vi "OpenGDSLicense_ProductInfo.vi"(5 "error in (no error)":errorcluster) -> (19 "error out":errorcluster)   [LabVIEW 2012]
uses:
  <resource>/Framework/Providers/Open_GDS/ClassProviders/Provider_EndevoGOOP300/ClassWriterGOOP300_class/ClassWriterGOOP300.lvclass
  <resource>/Framework/Providers/Open_GDS/ClassProviders/Provider_LvNativeClass/ClassWriterNative_class/ClassWriterNative.lvclass
  <resource>/Framework/Providers/Open_GDS/ClassProviders/Provider_EndevoGOOP400/ClassWriterGOOP400_class/ClassWriterGOOP400.lvclass
  <vilib>/event_ctls.llb/lveventtype.ctl
  <resource>/Framework/Providers/Open_GDS/SubVIs/GOOP_ToolVersion.vi
  <vilib>/Platform/browser.llb/Open URL in Default Browser (string).vi
panel:
  out "SwCheck":string
  in  "_GDSOnline":bool
  in  "_MainHelp":bool
  in  "_UnInstall":bool
  out "_Version":string="4.1  (Q3U)" caption="Version"
  in  "_OK":bool
  # "Open GOOP\nDevelopment Suite"
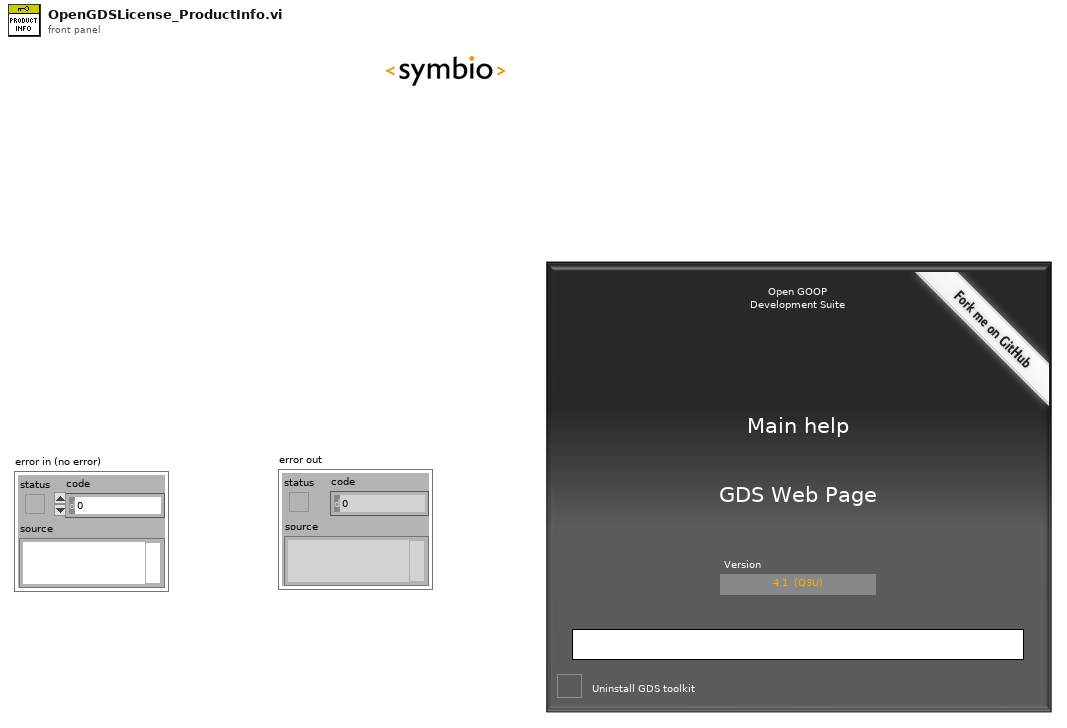
[diagram p1: front panel]
types:
  T1 = cluster{"Templates":path[], "TemplatesVersions":string[], "KernelVIs":path[], "KernelVersions":string[]}
  T2 = enum32{"None", "Stop", "Question", "Exclamation", "Information"}
  T3 = typedef "lveventtype.ctl" = enum32{"Null", "Timeout", "Annotation Menu Selection", "Annotation Menu Selection?", "App Instance Close", "App Instance Close?", "Autoscale Range Change", "Cell Edit", "Cell Edit?", "Cursor Grab", "Cursor Grab?", "Cursor Menu Selection", "Cursor Menu Selection?", "Cursor Move", "Cursor Release", "Data Change", "Direction Change", "Display State Change", "Drag Ended", "Drag Enter", "Drag Leave", "Drag Over", "Drag Source Update", "Drag Starting", "Drag Starting?", "Drop", "Exec State Change", "Key Down", "Key Down?", "Key Repeat", "Key Repeat?", "Key Up", "Listbox Double Click", "Menu Activation?", "Menu Selection (App)", "Menu Selection? (App)", "Menu Selection (User)", "Mouse Down", "Mouse Down?", "Mouse Enter", "Mouse Leave", "Mouse Move", "Mouse Up", "NI Security User Change (App)", "Pane Size", "Panel Close", "Panel Close?", "Panel Resize", "Plot Attribute Change", "Scale Range Change", "Shortcut Menu Activation?", "Shortcut Menu Selection (App)", "Shortcut Menu Selection? (App)", "Shortcut Menu Selection (User)", "Tree Double Click", "Tree Drag", "Tree Drag?", "Tree Drop", "Tree Drop?", "Tree Item Close", "Tree Item Close?", "Tree Item Open", "Tree Item Open?", "Value Change"}
  T4 = cluster{"Major":u16, "Minor":u16, "Fix":u16, "Build":u16}
  T5 = typedef "Librarian File List.ctl" = cluster{"name":string, "create date":u32, "mod date":u32, "type":string, "creator":string, "LV version":i32}[]
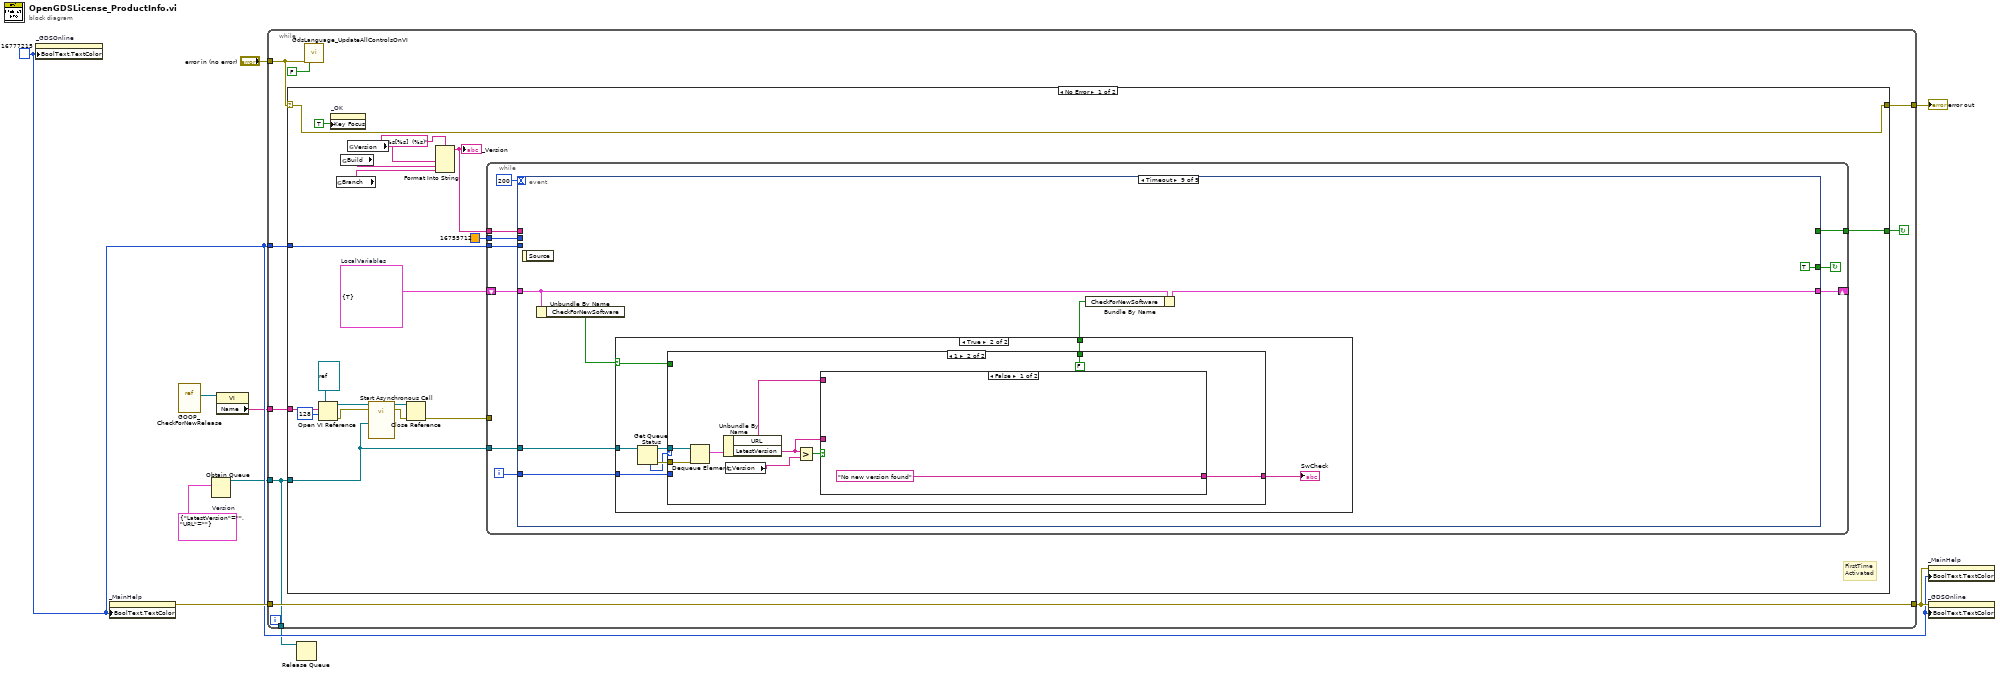
[diagram p0: block diagram]
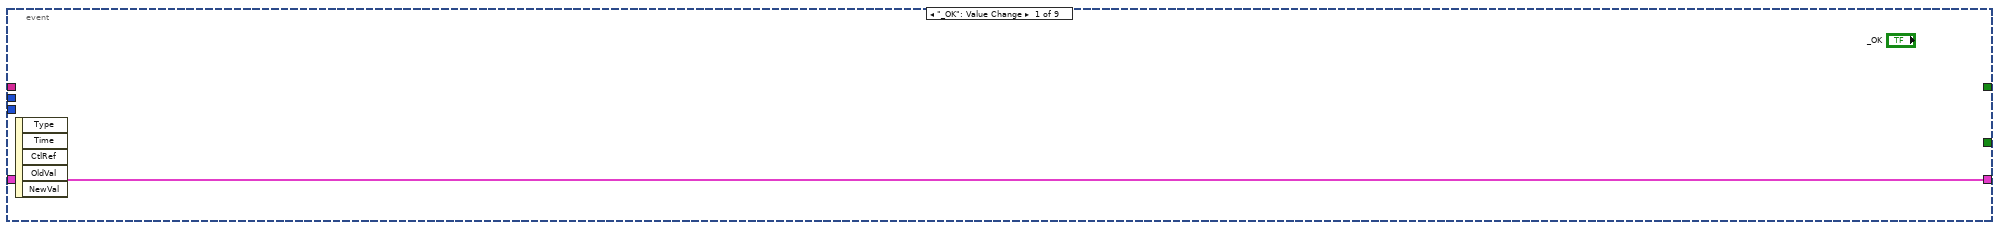
[diagram p2: hidden frame]
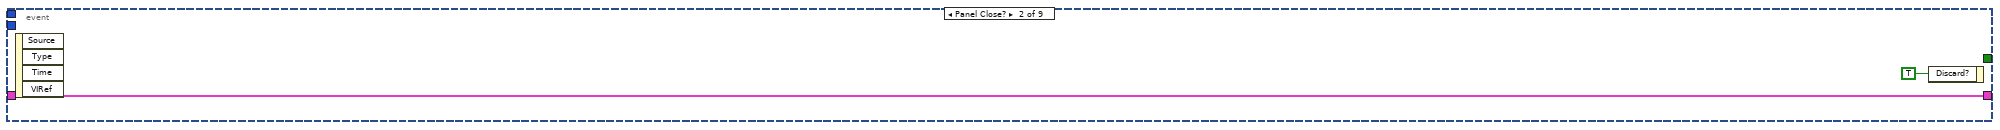
[diagram p3: hidden frame]
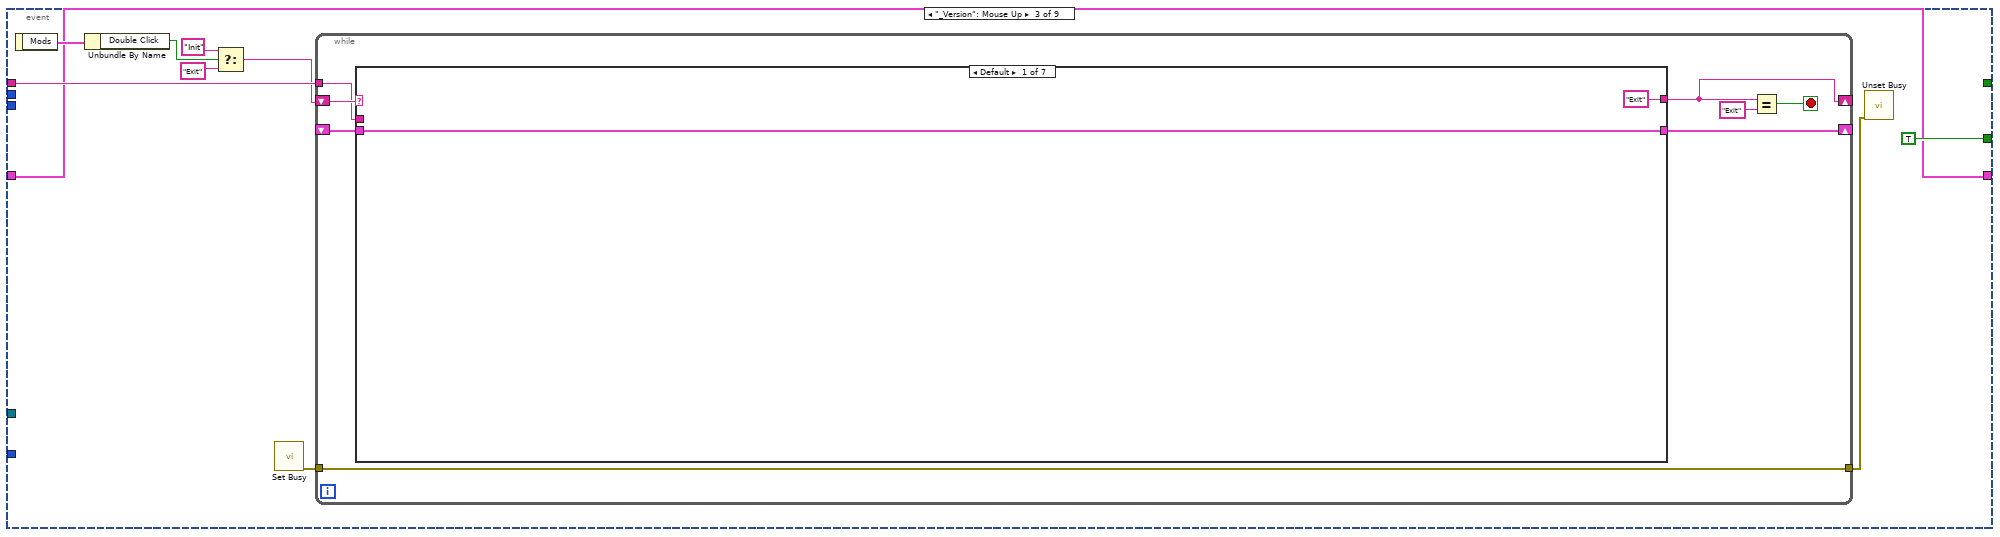
[diagram p4: hidden frame]
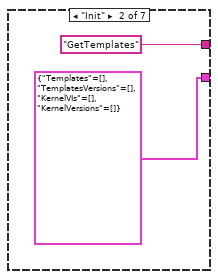
[diagram p5: hidden frame]
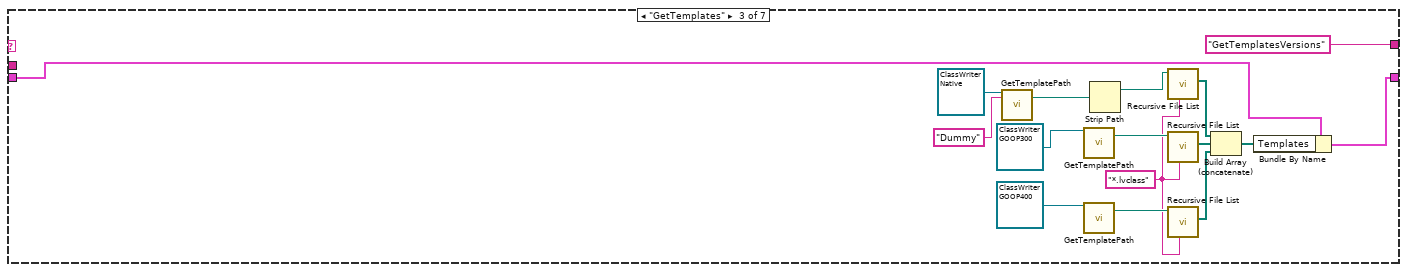
[diagram p6: hidden frame]
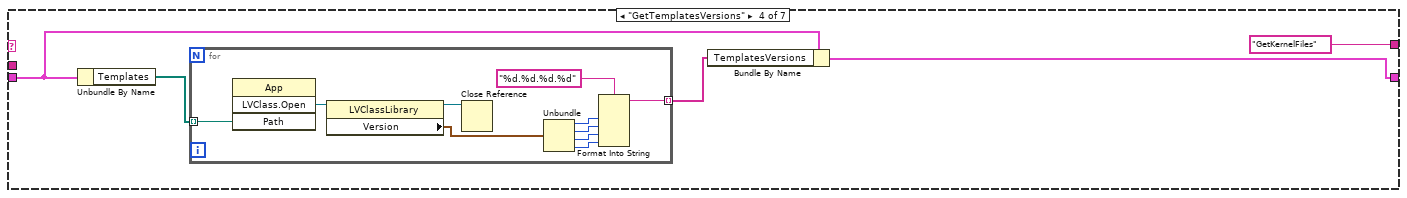
[diagram p7: hidden frame]
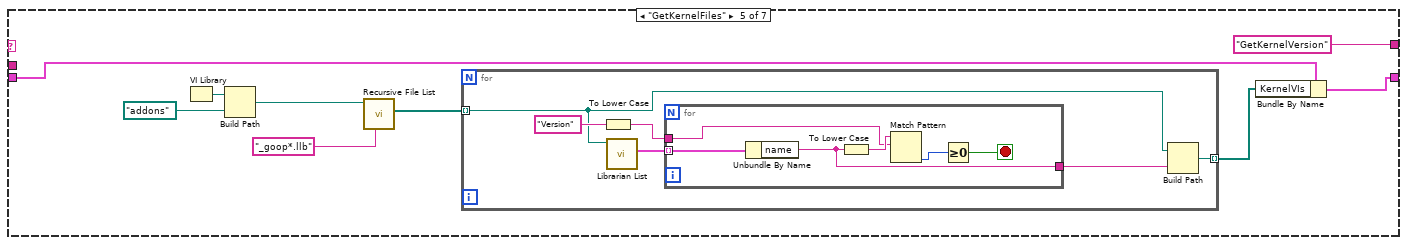
[diagram p8: hidden frame]
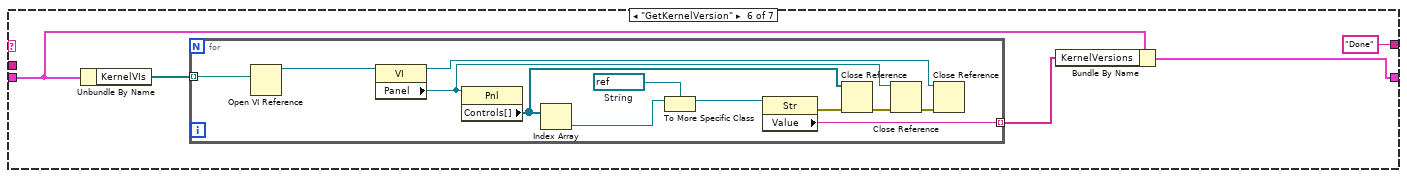
[diagram p9: hidden frame]
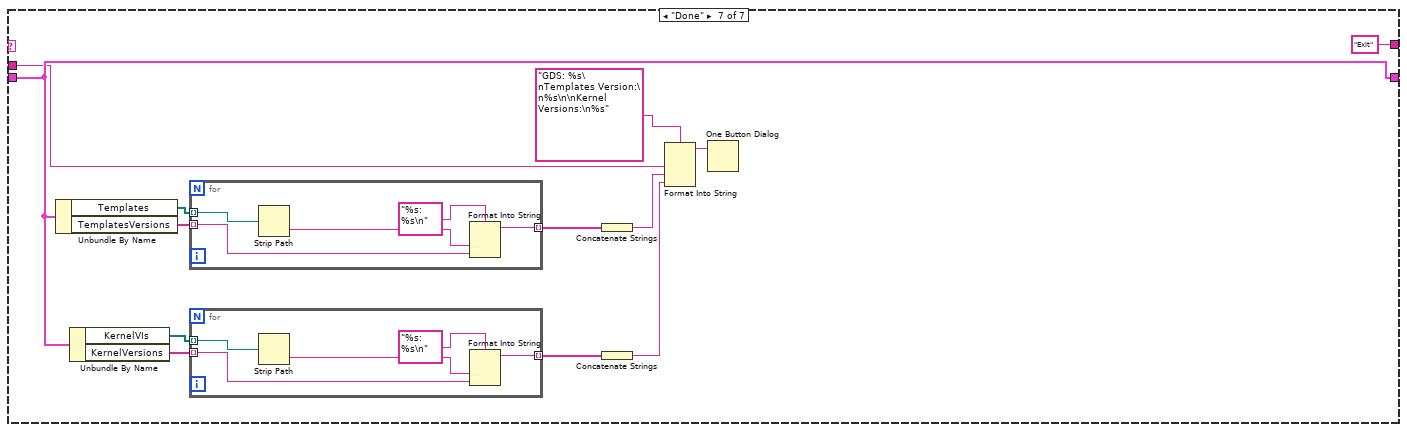
[diagram p10: hidden frame]
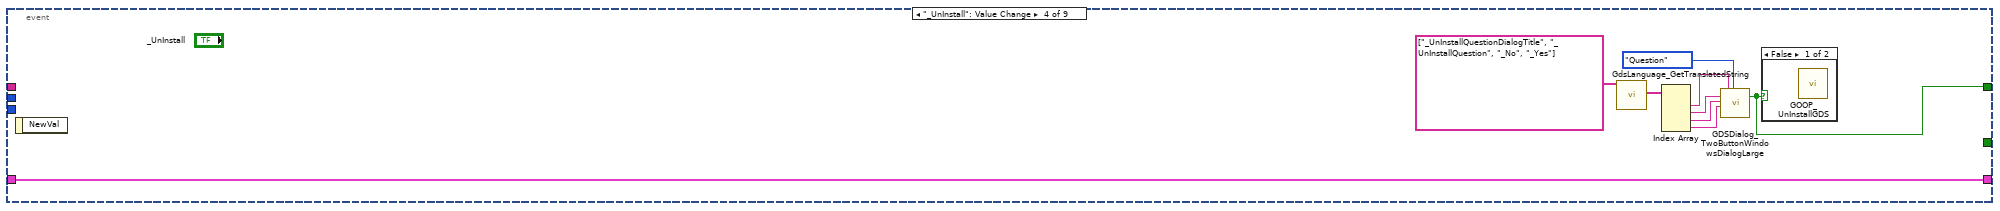
[diagram p11: hidden frame]
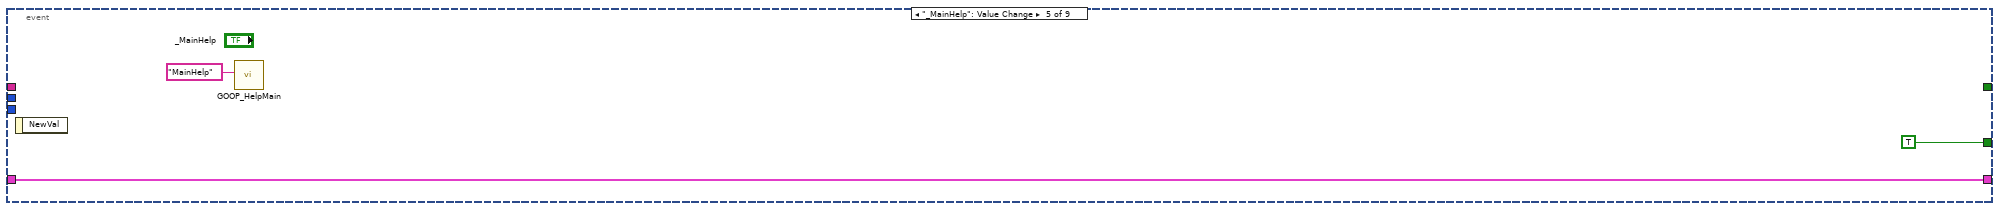
[diagram p13: hidden frame]
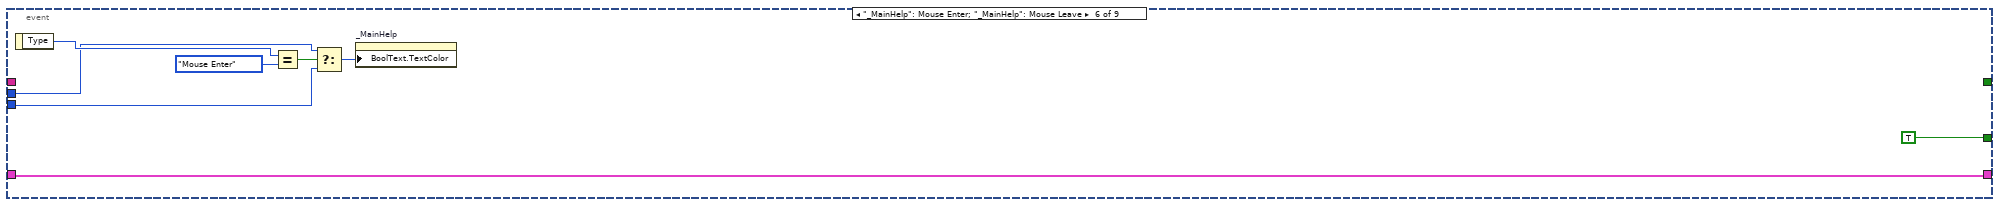
[diagram p14: hidden frame]
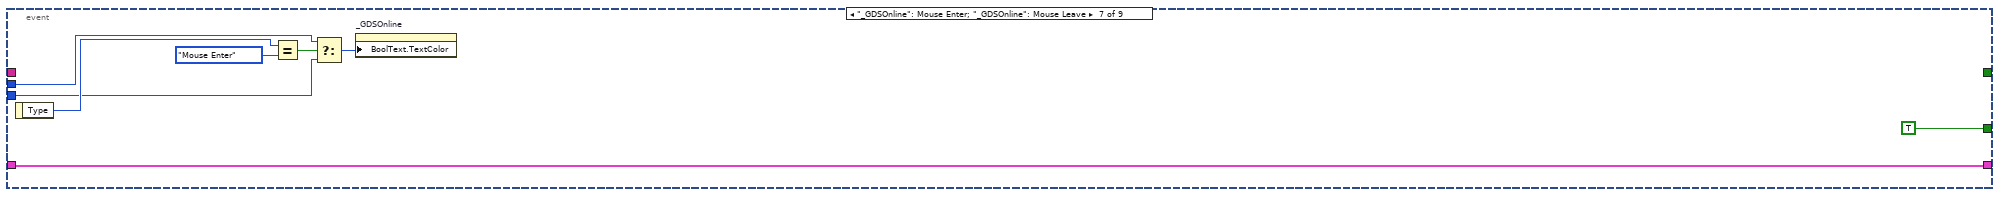
[diagram p15: hidden frame]
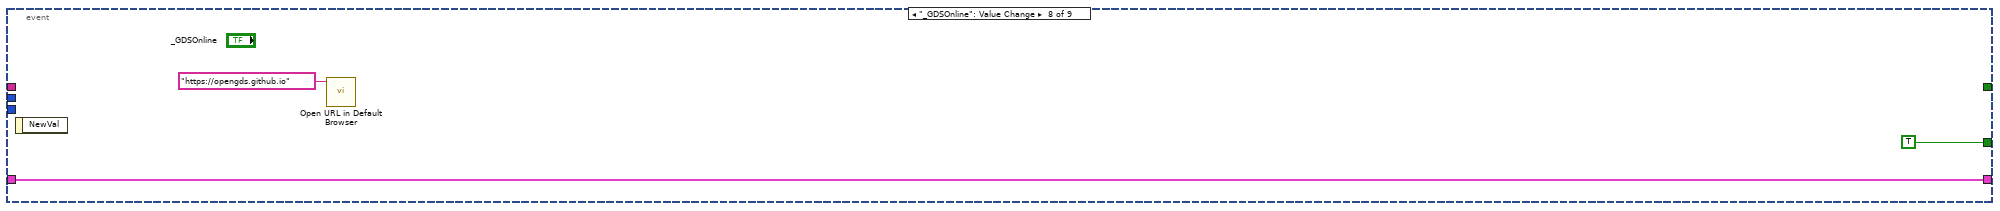
[diagram p16: hidden frame]
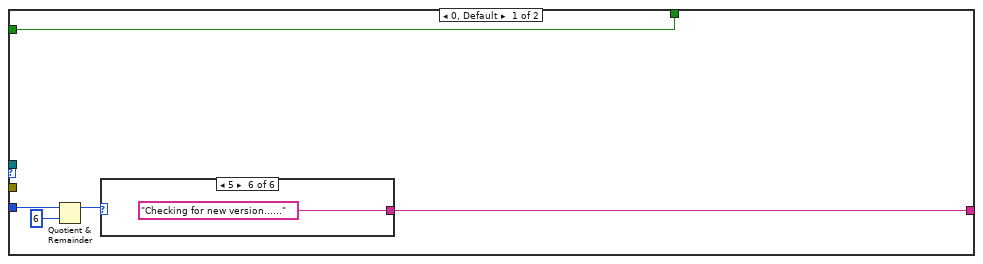
[diagram p18: hidden frame]
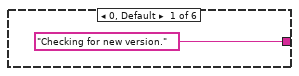
[diagram p19: hidden frame]
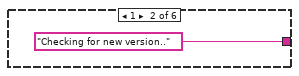
[diagram p20: hidden frame]
diagram:
  w3 = cluster{"LatestVersion":string, "URL":string} {"LatestVersion"="", "URL"=""}  # Version
  w6 = u32 16777215
  n1 = property on="_GDSOnline" class="Bool"("BoolText.TextColor"=w6) -> ()  [unwired: 2 in, 2 out]
  n2 = property on="_MainHelp" class="Bool"("BoolText.TextColor"=w6) -> (error out=w8:errorcluster)  [unwired: 2 in, 1 out]
  n3 = vi-ref <resource>:"GOOP_CheckForNewRelease.vi"() -> (w5:refnum<vi>)
  n4 = Obtain Queue(element data type=w3) -> (queue out=w2:refnum<queue>)  [unwired: 4 in, 2 out]
  n5 = property class="VI"(reference=w5) -> ("Name"=w4:string)  [unwired: 1 in, 2 out]
  n6 = while {
    tunnel: [w18] -> w10
    tunnel: "error in (no error)" -> [w13]
    tunnel: [w15] -> w7
    tunnel: w8 -> [w15]
    tunnel: w6 -> [w14]
    tunnel: w4 -> [w12]
    tunnel: w2 -> [w11]
    tunnel: [w11] -> w1
    stop <- w16 continue-if-true
    n7 = case shown="No Error" w13 {
      selector: w13 -> [w38 w244]
      tunnel: [w38 w244] -> w18
      tunnel: [w37 _] -> w16
      tunnel: w14 -> [w36 _]
      tunnel: w12 -> [w30 _]
      tunnel: w11 -> [w21 _]
      frame No Error {
        w26 = cluster{"CheckForNewSoftware":bool} {"CheckForNewSoftware"=TRUE}  # LocalVariables
        # "FirstTime\nActivated"
        n8 = Open VI Reference(type specifier VI Refnum (for type only)=refnum<vi> refnum, vi path=w30, options=128) -> (vi reference=w29:refnum<vi>, error out=w28:errorcluster)  [unwired: 3 in]
        n9 = property on="_OK" class="Bool"("Key Focus"=TRUE) -> ()  [unwired: 2 in, 2 out]
        n10 = global read "GOOP_ToolVersion.vi" "Branch"() -> (w20:string)
        n11 = global read "GOOP_ToolVersion.vi" "Build"() -> (w19:string)
        n12 = global read "GOOP_ToolVersion.vi" "Version"() -> (w35:string)
        n13 = call-by-ref "Start Asynchronous Call"(reference=w29, error in=w28, "QueueRef"=w21) -> (reference out=w24:refnum<vi>, error out=w23:errorcluster)  [unwired: 11 in]
        n14 = Close Reference(reference=w24, error in (no error)=w23) -> (error out=w22:errorcluster)
        n15 = Format Into String(format string="%s[%s]  (%s)", w35, w19, w20) -> (resulting string=w33:string)  [unwired: 2 in, 1 out]
        "_Version" <- w33
        n16 = while {
          tunnel: [w48] -> w37
          tunnel: w33 -> [w47]
          tunnel: u32 16755712 -> [w45]
          tunnel: w36 -> [w44]
          shift-right: [w41] -> _
          shift-left: w26 -> [w42]
          tunnel: w21 -> [w40]
          tunnel: w22 -> [_]
          i -> [w39]
          stop <- w46 continue-if-true
          n17 = event shown="[8] Timeout" {
            selector: _ -> [_ _ _ _ _ _ _ _ _]
            dyn-events: _ -> [_ _ _ _ _ _ _ _ _]
            timeout: 200 -> [_ _ _ _ _ _ _ _ _]
            tunnel: [_ _ _ w167 _ _ _ _ _] -> w48
            tunnel: w47 -> [_ _ w58 _ _ _ _ _ _]
            tunnel: [_ _ TRUE _ TRUE TRUE TRUE TRUE TRUE] -> w46
            tunnel: w45 -> [_ _ _ _ _ w180 w188 _ _]
            tunnel: w44 -> [_ _ _ _ _ w179 w187 _ _]
            tunnel: w42 -> [w49 w50 w52 w166 w175 w178 w186 w194 w203]
            tunnel: [w49 w50 w52 w166 w175 w178 w186 w194 w198] -> w41
            tunnel: w40 -> [_ _ _ _ _ _ _ _ w201]
            tunnel: w39 -> [_ _ _ _ _ _ _ _ w200]
            event "_OK": Value Change {
              n18 = event-data() -> ()  [unwired: 1 in, 5 out]
            }
            event Panel Close? {
              n19 = event-data() -> ()  [unwired: 1 in, 4 out]
              n20 = event-data("Discard?"=TRUE) -> ()  [unwired: 1 in, 1 out]
            }
            event "_Version": Mouse Up {
              n21 = event-data() -> ("Mods"=w61:cluster{"Double Click":bool, "Menu Key":bool})  [unwired: 1 in]
              n22 = Unbundle By Name(w61) -> ("Double Click"=w57:bool)
              n23 = Select(t="Init", s=w57, f="Exit") -> (s? t:f=w54:string)
              n24 = call <vilib>:"Set Busy.vi"() -> ("error out"=w60:errorcluster)  [unwired: 10 in, 1 out]
              n25 = while {
                shift-right: [w64] -> _
                shift-left: w54 -> [w69]
                shift-right: [w66] -> _
                shift-left: _ -> [w65]
                tunnel: w60 -> [w63]
                tunnel: [w63] -> w59
                tunnel: w58 -> [w62]
                stop <- w68 stop-if-true
                n26 = case shown="Default" w69 {
                  tunnel: ["Exit" "GetTemplates" "GetTemplatesVersions" "GetKernelFiles" "GetKernelVersion" "Done" "Exit"] -> w64
                  tunnel: [w70 T1 {"Templates"=[], "TemplatesVersions"=[], "KernelVIs"=[], "KernelVersions"=[]} w83 w91 w106 w127 w145] -> w66
                  tunnel: w65 -> [w70 _ w84 w93 w108 w129 w145]
                  tunnel: w62 -> [_ _ _ _ _ _ w143]
                  frame Default {
                  }
                  frame "Init" {
                  }
                  frame "GetTemplates" {
                    w77 = "*.lvclass" ("pattern")
                    n27 = call-dynamic "GetTemplatePath.vi"("reference in"=refnum<class "ClassWriterNative.lvclass"> refnum, "ClassTemplateSubDirectory"="Dummy") -> ("FolderPathOut"=w75:path)  [unwired: 14 in, 3 out]
                    n28 = call-dynamic "GetTemplatePath.vi"("reference in"=refnum<class "ClassWriterGOOP300.lvclass"> refnum) -> ("FolderPathOut"=w82:path)  [unwired: 15 in, 3 out]
                    n29 = call-dynamic "GetTemplatePath.vi"("reference in"=refnum<class "ClassWriterGOOP400.lvclass"> refnum ("ClassWriterGOOP400.lvclass")) -> ("FolderPathOut"=w80:path)  [unwired: 15 in, 3 out]
                    n30 = Strip Path(path=w75) -> (stripped path=w74:path)  [unwired: 1 out]
                    n31 = call <vilib>:"Recursive File List.vi"("pattern"=w77, "Folder Path"=w74) -> ("All Files in Dir"=w86:path[])  [unwired: 5 in, 4 out]
                    n32 = call <vilib>:"Recursive File List.vi"("pattern"=w77, "Folder Path"=w82) -> ("All Files in Dir"=w81:path[])  [unwired: 5 in, 4 out]
                    n33 = call <vilib>:"Recursive File List.vi"("pattern"=w77, "Folder Path"=w80) -> ("All Files in Dir"=w79:path[])  [unwired: 5 in, 4 out]
                    n34 = Build Array (concatenate)(w86, w81, w79) -> (w85:path[])
                    n35 = Bundle By Name(cluster=w84, "Templates"=w85) -> (w83:T1)
                  }
                  frame "GetTemplatesVersions" {
                    n36 = Unbundle By Name(w93) -> ("Templates"=w94:path[])
                    n37 = for {
                      tunnel: w94 -> [w104] mode=indexing
                      tunnel: [w96] -> w92 mode=indexing
                      n38 = invoke class="App" method="LVClass.Open"("Path"=w104) -> ("LVClass.Open"=w103:refnum<vi>)  [unwired: 3 in, 3 out]
                      n39 = property class="LVClassLibrary"(reference=w103) -> (reference out=w95:refnum<vi>, "Version"=w102:T4)  [unwired: 1 in, 1 out]
                      n40 = Close Reference(reference=w95) -> ()  [unwired: 1 in, 1 out]
                      n41 = Unbundle(w102) -> ("Major"=w100:u16, "Minor"=w99:u16, "Fix"=w98:u16, "Build"=w97:u16)
                      n42 = Format Into String(format string="%d.%d.%d.%d", w100, w99, w98, w97) -> (resulting string=w96:string)  [unwired: 2 in, 1 out]
                    }
                    n43 = Bundle By Name(cluster=w93, "TemplatesVersions"=w92) -> (w91:T1)
                  }
                  frame "GetKernelFiles" {
                    n44 = VI Library() -> (path=w113:path)
                    n45 = Build Path(base path=w113, name or relative path=path "addons") -> (appended path=w111:path)
                    n46 = call <vilib>:"Recursive File List.vi"("pattern"="_goop*.llb", "Folder Path"=w111) -> ("All Files in Dir"=w109:path[])  [unwired: 5 in, 4 out]
                    n47 = for {
                      tunnel: w109 -> [w115] mode=indexing
                      tunnel: [w114] -> w107 mode=indexing
                      n48 = To Lower Case(string="Version" ("regular expression")) -> (all lower case string=w117:string)
                      n49 = call <vilib>:"Librarian List.vi"("path"=w115) -> ("file list"=w119:T5)  [unwired: 9 in, 1 out]
                      n50 = for {
                        tunnel: w119 -> [w125] mode=indexing
                        tunnel: w117 -> [w123]
                        tunnel: [w120] -> w116
                        stop <- w121 stop-if-true
                        n51 = Unbundle By Name(w125) -> ("name"=w120:string)
                        n52 = To Lower Case(string=w120) -> (all lower case string=w124:string)
                        n53 = Match Pattern(string=w124, regular expression=w123) -> (offset past match=w122:i32)  [unwired: 1 in, 3 out]
                        n54 = Greater Or Equal To 0?(x=w122) -> (x >= 0?=w121:bool)
                      }
                      n55 = Build Path(base path=w115, name or relative path=w116) -> (appended path=w114:path)
                    }
                    n56 = Bundle By Name(cluster=w108, "KernelVIs"=w107) -> (w106:T1)
                  }
                  frame "GetKernelVersion" {
                    n57 = Unbundle By Name(w129) -> ("KernelVIs"=w130:path[])
                    n58 = for {
                      tunnel: w130 -> [w142] mode=indexing
                      tunnel: [w137] -> w128 mode=indexing
                      w139 = refnum<vi> refnum  # String
                      n59 = Open VI Reference(vi path=w142) -> (vi reference=w141:refnum<vi>)  [unwired: 5 in, 1 out]
                      n60 = property class="VI"(reference=w141) -> (reference out=w131:refnum<vi>, "Panel"=w133:refnum<vi>)  [unwired: 1 in, 1 out]
                      n61 = property class="Pnl"(reference=w133) -> ("Controls[]"=w135:refnum<vi>[])  [unwired: 1 in, 2 out]
                      n62 = Index Array(array=w135) -> (element=w140:refnum<vi>)  [unwired: 1 in]
                      n63 = To More Specific Class(target class=w139, reference=w140) -> (specific class reference=w138:refnum<vi>)  [unwired: 1 in, 1 out]
                      n64 = property class="Str"(reference=w138) -> (error out=w136:errorcluster, "Value"=w137:string)  [unwired: 1 in, 1 out]
                      n65 = Close Reference(reference=w135, error in (no error)=w136) -> (error out=w134:errorcluster)
                      n66 = Close Reference(reference=w133, error in (no error)=w134) -> (error out=w132:errorcluster)
                      n67 = Close Reference(reference=w131, error in (no error)=w132) -> ()  [unwired: 1 out]
                    }
                    n68 = Bundle By Name(cluster=w129, "KernelVersions"=w128) -> (w127:T1)
                  }
                  frame "Done" {
                    n69 = Unbundle By Name(w145) -> ("Templates"=w155:path[], "TemplatesVersions"=w154:string[])
                    n70 = Unbundle By Name(w145) -> ("KernelVIs"=w150:path[], "KernelVersions"=w151:string[])
                    n71 = for {
                      tunnel: w155 -> [w165] mode=indexing
                      tunnel: w154 -> [w162] mode=indexing
                      tunnel: [w161] -> w153 mode=indexing
                      n72 = Strip Path(path=w165) -> (name=w163:string)  [unwired: 1 out]
                      n73 = Format Into String(format string="%s: %s\n", w163, w162) -> (resulting string=w161:string)  [unwired: 2 in, 1 out]
                    }
                    n74 = for {
                      tunnel: w150 -> [w160] mode=indexing
                      tunnel: w151 -> [w157] mode=indexing
                      tunnel: [w156] -> w152 mode=indexing
                      n75 = Strip Path(path=w160) -> (name=w158:string)  [unwired: 1 out]
                      n76 = Format Into String(format string="%s: %s\n", w158, w157) -> (resulting string=w156:string)  [unwired: 2 in, 1 out]
                    }
                    n77 = Concatenate Strings(w153) -> (w148:string)
                    n78 = Concatenate Strings(w152) -> (w147:string)
                    n79 = Format Into String(format string="GDS: %s\nTemplates Version:\n%s\n\nKernel Versions:\n%s", w143, w148, w147) -> (resulting string=w146:string)  [unwired: 2 in, 1 out]
                    n80 = One Button Dialog(message=w146) -> ()  [unwired: 1 in, 1 out]
                  }
                }
                n81 = Equal?(x=w64, y="Exit") -> (x = y?=w68:bool)
              }
              n82 = call <vilib>:"Unset Busy.vi"("error in (no error)"=w59) -> ()  [unwired: 10 in, 1 out]
            }
            event "_UnInstall": Value Change {
              n83 = event-data() -> ()  [unwired: 1 in, 1 out]
              n84 = call <resource>:"GdsLanguage_GetTranslatedString.vi"("StringID(s)"=string[] ["_UnInstallQuestionDialogTitle", "_UnInstallQuestion", "_No", "_Yes"]) -> ("StringsOut"=w169:string[])  [unwired: 15 in, 3 out]
              n85 = Index Array(array=w169) -> (element #1=w171:string, element #2=w168:string, element #3=w173:string, element #4=w172:string)  [unwired: 4 in]
              n86 = call <resource>:"GDSDialog_TwoButtonWindowsDialogLarge.vi"("UserText"=w168, "Button1Name"=w173, "Button2Name"=w172, "DialogTitle"=w171, "Icon"=T2."Question") -> ("Button1Pressed"=w167:bool)  [unwired: 12 in, 2 out]
              n87 = case shown="False" w167 {
                frame False {
                  n88 = call <resource>:"GOOP_UnInstallGDS.vi"() -> ()  [unwired: 19 in, 1 out]
                }
                frame True {
                }
              }
            }
            event "_MainHelp": Value Change {
              n89 = event-data() -> ()  [unwired: 1 in, 1 out]
              n90 = call <resource>:"GOOP_HelpMain.vi"("File"="MainHelp") -> ()  [unwired: 11 in]
            }
            event "_MainHelp": Mouse Enter; "_MainHelp": Mouse Leave {
              n91 = event-data() -> ("Type"=w185:T3)  [unwired: 1 in]
              n92 = Equal?(x=w185, y=lveventtype."Mouse Enter") -> (x = y?=w183:bool)
              n93 = Select(t=w180, s=w183, f=w179) -> (s? t:f=w182:u32)
              n94 = property on="_MainHelp" class="Bool"("BoolText.TextColor"=w182) -> ()  [unwired: 2 in, 2 out]
            }
            event "_GDSOnline": Mouse Enter; "_GDSOnline": Mouse Leave {
              n95 = event-data() -> ("Type"=w193:T3)  [unwired: 1 in]
              n96 = Equal?(x=w193, y=lveventtype."Mouse Enter") -> (x = y?=w191:bool)
              n97 = Select(t=w188, s=w191, f=w187) -> (s? t:f=w190:u32)
              n98 = property on="_GDSOnline" class="Bool"("BoolText.TextColor"=w190) -> ()  [unwired: 2 in, 2 out]
            }
            event "_GDSOnline": Value Change {
              n99 = event-data() -> ()  [unwired: 1 in, 1 out]
              n100 = call-poly <vilib>:"Open URL in Default Browser.vi"("URL"="https://opengds.github.io") -> ()  [unwired: 5 in, 2 out]
            }
            event Timeout {
              n101 = event-data() -> ()  [unwired: 1 in, 1 out]
              n102 = Unbundle By Name(w203) -> ("CheckForNewSoftware"=w202:bool)
              n103 = case shown="True" w202 {
                selector: w202 -> [w204 w207]
                tunnel: w201 -> [_ w212]
                tunnel: w200 -> [_ w211]
                tunnel: [w204 w206] -> w197
                frame False {
                }
                frame True {
                  n104 = Get Queue Status(queue=w212) -> (queue out=w210:refnum<queue>, error out=w209:errorcluster, # elements in queue=w205:i32)  [unwired: 2 in, 5 out]
                  n105 = case shown="1" w205 {
                    tunnel: w211 -> [w217 _]
                    tunnel: w210 -> [_ w232]
                    tunnel: w209 -> [_ w231]
                    tunnel: [w214 w227] -> w208
                    tunnel: w207 -> [w213 _]
                    tunnel: [w213 FALSE] -> w206
                    frame 0, Default {
                      n106 = Quotient & Remainder(x=w217, y=6) -> (x-y*floor(x/y)=w215:i32)  [unwired: 1 out]
                      n107 = case shown="5" w215 {
                        tunnel: ["Checking for new version." "Checking for new version.." "Checking for new version..." "Checking for new version...." "Checking for new version....." "Checking for new version......"] -> w214
                        frame 0, Default {
                        }
                        frame 1 {
                        }
                        frame 2 {
                        }
                        frame 3 {
                        }
                        frame 4 {
                        }
                        frame 5 {
                        }
                      }
                    }
                    frame 1 {
                      n108 = Dequeue Element(queue=w232, error in (no error)=w231) -> (element=w230:cluster{"LatestVersion":string, "URL":string})  [unwired: 1 in, 3 out]
                      n109 = Unbundle By Name(w230) -> ("URL"=w225:string, "LatestVersion"=w226:string)
                      n110 = global read "GOOP_ToolVersion.vi" "Version"() -> (w229:string)
                      n111 = Greater?(x=w226, y=w229) -> (0:w228:bool)
                      n112 = case shown="False" w228 {
                        tunnel: ["No new version found" w241] -> w227
                        tunnel: w226 -> [_ w239]
                        tunnel: w225 -> [_ w235]
                        frame False {
                        }
                        frame True {
                          n113 = Format Into String(format string="New version found: %s\nDo you want to start downlaoding that version now?", w239) -> (resulting string=w238:string)  [unwired: 2 in, 1 out]
                          n114 = Format Into String(format string="New version found: %s", w239) -> (resulting string=w241:string)  [unwired: 2 in, 1 out]
                          n115 = Two Button Dialog(message=w238, 1:"No" ("F button name (\"Cancel\")"), 2:"Yes" ("T button name (\"OK\")")) -> (T button?=w234:bool)
                          n116 = case shown="True" w234 {
                            tunnel: w235 -> [_ w243]
                            frame False {
                            }
                            frame True {
                              n117 = call-poly <vilib>:"Open URL in Default Browser.vi"("URL"=w243) -> ()  [unwired: 5 in, 2 out]
                            }
                          }
                        }
                      }
                    }
                  }
                  "SwCheck" <- w208
                }
              }
              n118 = Bundle By Name(cluster=w203, "CheckForNewSoftware"=w197) -> (w198:cluster{"CheckForNewSoftware":bool})
            }
          }
        }
      }
      frame Error {
      }
    }
    n119 = call <resource>:"GdsLanguage_UpdateAllControlsOnVI.vi"("error in (no error)"=w13, "CreateLanguageFile(Use this to create a languageFile)"=FALSE) -> ()  [unwired: 16 in, 2 out]
  }
  "error out" <- w10
  n120 = Release Queue(queue=w1) -> ()  [unwired: 2 in, 3 out]
  n121 = property on="_MainHelp" class="Bool"(error in=w7, "BoolText.TextColor"=w6) -> ()  [unwired: 1 in, 2 out]
  n122 = property on="_GDSOnline" class="Bool"(error in=w7, "BoolText.TextColor"=w6) -> ()  [unwired: 1 in, 2 out]
